vi "Binary_SpectroscopyFile-Plot3D-Surface.vi"() -> ()   [LabVIEW 2021]
doc: "<B>This example uses the \"3D Parametric Graph\" to display a 3D view of the surface.</B>\n\nOpens a binary file, reads the parameters of each spectroscopy experiment, extracts the Z (m) parameter (topography data) and displays the topography data in a 3D display.\n\n- Nanonis Programming Interface -"
uses:
  Nanonis Prog Interface.lvlib
  <vilib>/Platform/NI_3dgraph.lvlib
panel:
  in  "3D Parametric Surface":refnum<k7>(container)
  out "error out":errorcluster
  in  "Binary Spectroscopy File":path
  # "This example uses the \"3D Parametric Graph\" to display a 3D view of the surface"
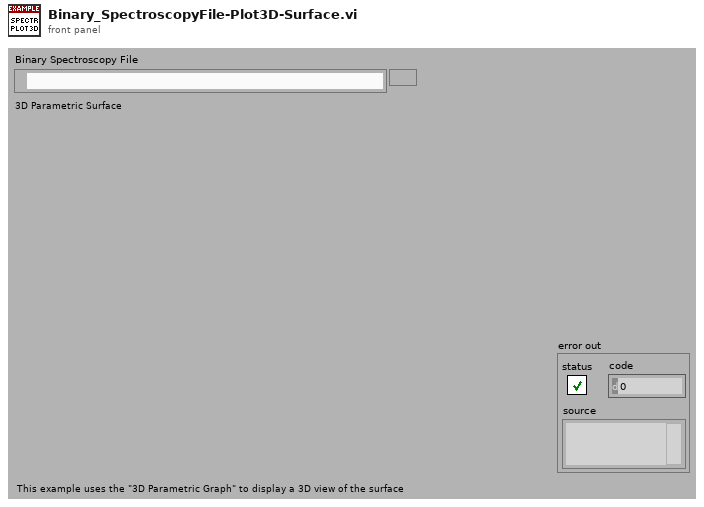
[diagram p1: front panel]
types:
  T1 = typedef "Nanonis Prog Interface.lvlib/Binary_SpectroscopyFile-Config.ctl" = cluster{"Num Par":i32, "Exp size":i32, "Points":i32, "Grid Dim X":i32, "Grid Dim Y":i32, "Header size":i32, "Channels":string[], "Parameters":string[], "Sweep Signal":string, "Grid":cluster{"center X (m)":sgl, "center Y (m)":sgl, "width (m)":sgl, "height (m)":sgl, "angle (deg)":sgl}}
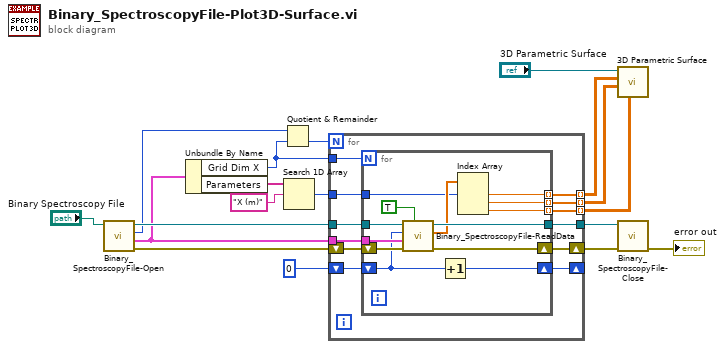
[diagram p0: block diagram]
diagram:
  n1 = call "Binary_SpectroscopyFile-Open.vi"("Binary Spectroscopy File"="Binary Spectroscopy File") -> ("error out"=w16:errorcluster, "Config"=w5:T1, "Number of Experiments"=w11:i32, "File ref"=w18:refnum<file>)  [unwired: 6 in, 1 out]
  n2 = Unbundle By Name(w5) -> ("Grid Dim X"=w4:i32, "Parameters"=w3:string[])
  n3 = Quotient & Remainder(x=w11, y=w4) -> (floor(x/y)=w10:i32)  [unwired: 1 out]
  n4 = Search 1D Array(1D array=w3, element="X (m)" ("string")) -> (index of element=w1:i32)  [unwired: 1 in]
  n5 = for {
    N: w10 -> [_]
    tunnel: w18 -> [w30]
    tunnel: w5 -> [w28]
    shift-right: [w27] -> w15
    shift-left: w16 -> [w29]
    tunnel: [w26] -> w14
    tunnel: w4 -> [w25]
    tunnel: [w24] -> w9 mode=indexing
    tunnel: [w23] -> w8 mode=indexing
    tunnel: [w22] -> w7 mode=indexing
    shift-right: [w20] -> _
    shift-left: 0 -> [w21]
    tunnel: w1 -> [w19]
    n6 = for {
      N: w25 -> [_]
      tunnel: w30 -> [w43]
      tunnel: w28 -> [w41]
      tunnel: [w38] -> w26
      shift-right: [w39] -> w27
      shift-left: w29 -> [w42]
      tunnel: [w36] -> w24 mode=indexing
      tunnel: [w35] -> w23 mode=indexing
      tunnel: [w34] -> w22 mode=indexing
      shift-right: [w32] -> w20
      shift-left: w21 -> [w33]
      tunnel: w19 -> [w31]
      n7 = call "Binary_SpectroscopyFile-ReadData.vi"("Read Parameters only? (F)"=TRUE, "error in"=w42, "Config"=w41, "Experiment to read (Index)"=w33, "File ref In"=w43) -> ("error out"=w39:errorcluster, "Parameter values"=w37:sgl[], "File ref Out"=w38:refnum<file>)  [unwired: 3 in, 1 out]
      n8 = Increment(x=w33) -> (x+1=w32:i32)
      n9 = Index Array(array=w37, index #1=w31) -> (element #1=w36:sgl, element #2=w35:sgl, element #3=w34:sgl)  [unwired: 2 in]
    }
  }
  n10 = call <vilib>:"3D Parametric Surface.vi"("z matrix"=w7, "y matrix"=w8, "x matrix"=w9, "3D graph"="3D Parametric Surface") -> ()  [unwired: 6 in, 2 out]
  n11 = call "Binary_SpectroscopyFile-Close.vi"("error in"=w15, "File ref"=w14) -> ("error out"=→"error out":errorcluster)  [unwired: 9 in]
